vi "modulation.vi"(7 "LWSR":refnum<class "Web Request.lvclass">, 11 "val":string) -> ()   [LabVIEW 2014]
uses:
  <vilib>/wsapi/Web Request.lvclass
  Instr Actor/Messages/Set Modulation MSG/Set Modulation MSG.lvclass
  Controller/Controls/Enqueuer Enum.ctl
  Instr Actor/Messages/Set Modulation MSG/Set Modulation MSG.lvclass/Set Modulation MSG.ctl
  Instr Actor/Messages/Set Modulation MSG/Write Modulation.vi
  Controller/Controller.lvclass
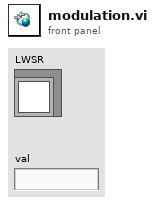
[diagram p1: front panel]
types:
  T1 = typedef "Enqueuer Enum.ctl" = enum8{"PAS", "CRDS", "File"}
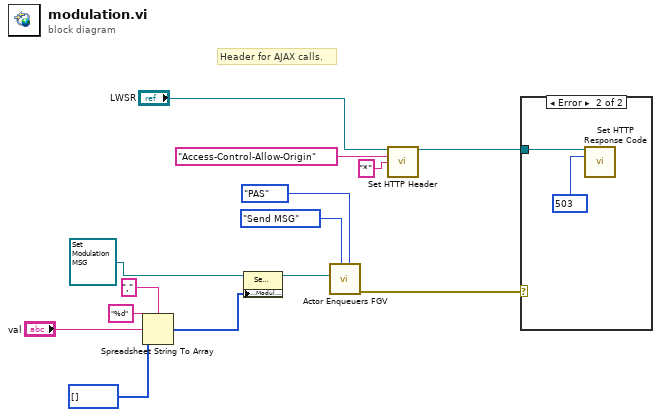
[diagram p0: block diagram]
diagram:
  # "Header for AJAX calls."
  n1 = Spreadsheet String To Array(delimiter (Tab)=",", format string="%d", spreadsheet string="val", array type (2D Dbl)=u8[] []) -> (array=w2:u8[])
  n2 = property class="Set Modulation MSG.lvclass"(reference=refnum<class "Set Modulation MSG.lvclass"> refnum ("ePAS Library.lvlib:Set Modulation MSG.lvclass"), "Accessors:Modulation"=w2) -> (reference out=w3:refnum<class "Set Modulation MSG.lvclass">)  [unwired: 1 in, 1 out]
  n3 = call "Actor Enqueuers FGV.vi"("Enqueuer"=Enqueuer_Enum."PAS", "State"=enum16{"Store", "Send MSG"}."Send MSG", "MSG"=w3) -> ("error out"=w5:errorcluster)  [unwired: 8 in]
  n4 = call <vilib>:"Set HTTP Header.vi"("LabVIEW Web Service Request"="LWSR", "header"="Access-Control-Allow-Origin", "header value"="*") -> ("LabVIEW Web Service Request out"=w6:refnum<class "Web Request.lvclass">)  [unwired: 11 in, 1 out]
  n5 = case shown="Error" w5 {
    tunnel: w6 -> [_ w15]
    frame No Error {
    }
    frame Error {
      w16 = 503 items=["100"=100, "101"=101, "200"=200, "201"=201, "202"=202, "203"=203, "204"=204, "205"=205, "206"=206, "300"=300, "301"=301, "302"=302, "303"=303, "304"=304, "305"=305, "306"=306, "307"=307, "400"=400, "401"=401, "402"=402, "403"=403, "404"=404, "405"=405, "406"=406, "407"=407, "408"=408, "409"=409, "410"=410, "411"=411, "412"=412, "413"=413, "414"=414, "415"=415, "416"=416, "417"=417, "500"=500, "501"=501, "502"=502, "503"=503, "504"=504, "505"=505] ("response code (200)")
      n6 = call <vilib>:"Set HTTP Response Code.vi"("LabVIEW Web Service Request"=w15, "response code (200)"=w16) -> ()  [unwired: 12 in, 2 out]
    }
  }
